vi "Get_PICAM_version.vi"(8 "error in":errorcluster) -> (0 "error out":errorcluster, 2 "PICam version":string)   [LabVIEW 2014, in "PICam.lvlib"]
doc: "Description\nPicam_GetVersion() returns PICam version information.\nThe following version information may be requested:\n• Major\nThis is the Major release version which is incremented with each major feature\naddition or breaks backward-compatibility.\n• Minor\nThis is the Minor release version which is incremented with minor feature\nadditions.\n• Distribution\nThis is the Distribution version which is incremented with bug fix releases.\n• Released\nThis is the date of the current official release in the format YYMM.\nWhen a release is classified as a Beta release, requesting this information returns a\nzero (0).\n\nNote: Picam_GetVersion() may be called prior to initializing the\nlibrary with Picam_InitializeLibrary()."
uses:
  PICam.lvlib
  Picam32.dll
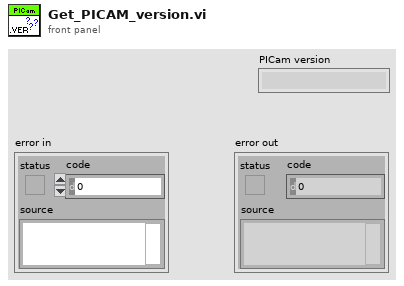
[diagram p1: front panel]
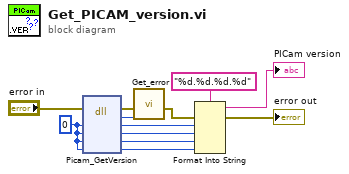
[diagram p0: block diagram]
diagram:
  w9 = 0 ("major")
  n1 = dll-call lib="Picam32.dll" fn="Picam_GetVersion"(error in="error in", "major"=w9, "minor"=w9, "distribution"=w9, "released"=w9) -> (error out=w11:errorcluster, "return type"=w10:i32, "major"=w5:i32, "minor"=w4:i32, "distribution"=w3:i32, "released"=w2:i32)  [unwired: 2 in, 1 out]
  n2 = call "Get_error.vi"("PICam_Error"=w10, "error in (no error)"=w11) -> ("error out"=w8:errorcluster)  [unwired: 9 in]
  n3 = Format Into String(format string="%d.%d.%d.%d", error in=w8, w5, w4, w3, w2) -> (resulting string=→"PICam version":string, error out=→"error out":errorcluster)  [unwired: 1 in]
